vi "LINC Insert Bit Stream.vi"(5 "little endian":bool, 6 "data to insert":string="\u0003", 7 "bit size":i32=2, 8 "bit offset":i32=16, 9 "data in":string="\u0000\u0000\u0000\u0000\u0000\u0000\u0000\u0000\u0000\u0000\u0000\u0000\u0000\u0000\u0000\u0000\u0000\u0000") -> (1 "data out":string)   [LabVIEW 2018, in "STEPkgDriver_LINC.lvlib"]
uses:
  STEPkgDriver_LINC.lvlib
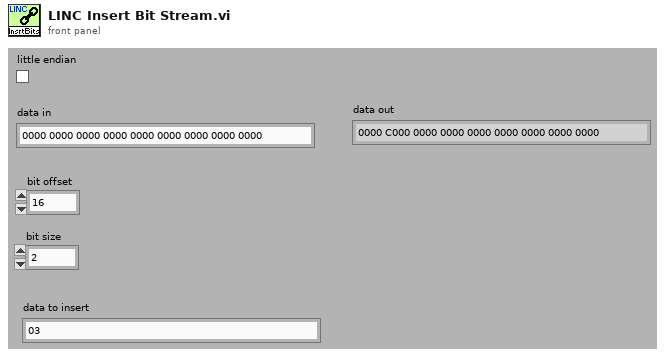
[diagram p1: front panel]
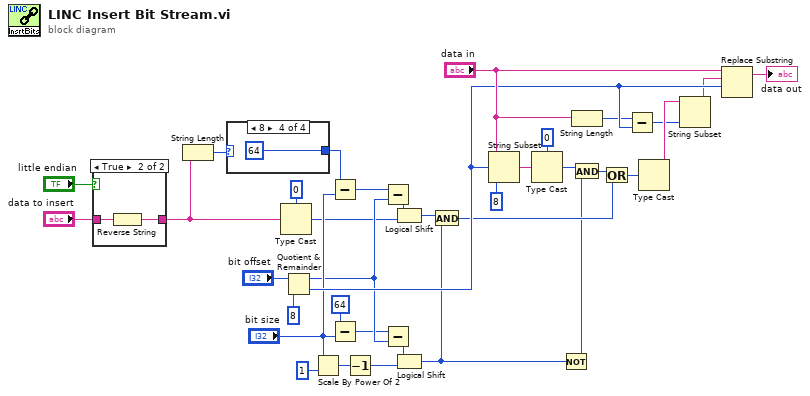
[diagram p0: block diagram]
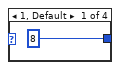
[diagram p2: hidden frame]
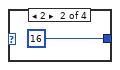
[diagram p3: hidden frame]
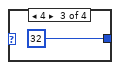
[diagram p4: hidden frame]
diagram:
  n1 = case shown="True" "little endian" {
    tunnel: "data to insert" -> [w37 w39]
    tunnel: [w37 w38] -> w27
    frame False {
    }
    frame True {
      n2 = Reverse String(1:w39) -> (0:w38:string)
    }
  }
  n3 = String Length(string=w27) -> (length=w25:i32)
  n4 = case shown="8" w25 {
    tunnel: [8 16 32 64] -> w6
    frame 1, Default {
    }
    frame 2 {
    }
    frame 4 {
    }
    frame 8 {
    }
  }
  n5 = Type Cast(type=u64 0, x=w27) -> (*(type *) &x=w26:u64)
  n6 = Quotient & Remainder(x="bit offset", y=8) -> (x-y*floor(x/y)=w30:i32, floor(x/y)=w32:i32)
  n7 = Scale By Power Of 2(n="bit size", x=u64 1) -> (x*2^n=w13:u64)
  n8 = Subtract(x=w6, y="bit size") -> (x-y=w5:i32)
  n9 = Subtract(x=64, y="bit size") -> (x-y=w2:i32)
  n10 = Decrement(x=w13) -> (x-1=w14:u64)
  n11 = Subtract(x=w5, y=w30) -> (x-y=w4:i32)
  n12 = Subtract(x=w2, y=w30) -> (x-y=w1:i32)
  n13 = Logical Shift(y=w4, x=w26) -> (x << y=w19:u64)
  n14 = Logical Shift(y=w1, x=w14) -> (x << y=w20:u64)
  n15 = And(x=w19, y=w20) -> (x .and. y?=w21:u64)
  n16 = String Subset(string="data in", offset (0)=w32, length (rest)=8 ("length (rest)")) -> (substring=w11:string)
  n17 = Type Cast(type=u64 0, x=w11) -> (*(type *) &x=w15:u64)
  n18 = Not(x=w20) -> (.not. x?=w16:u64)
  n19 = String Length(string="data in") -> (length=w8:i32)
  n20 = And(x=w15, y=w16) -> (x .and. y?=w17:u64)
  n21 = Or(x=w17, y=w21) -> (x .or. y?=w18:u64)
  n22 = Subtract(x=w8, y=w32) -> (x-y=w7:i32)
  n23 = Type Cast(x=w18) -> (*(type *) &x=w22:string)  [unwired: 1 in]
  n24 = String Subset(string=w22, length (rest)=w7) -> (substring=w23:string)  [unwired: 1 in]
  n25 = Replace Substring(3:w32, 4:w23, 5:"data in") -> (1:→"data out":string)  [unwired: 2 out]
